vi "Demap symbols.vi"(7 "Symbols":cdb[](array[numeric]) format="%.2f", 9 "Symbol Map":cdb[](array[numeric]) format="%.3f") -> (3 "Output Bit Stream":i8[](array[numeric]))   [LabVIEW 2011]
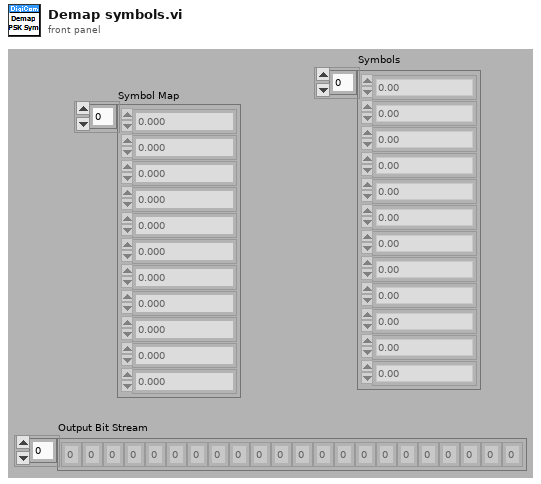
[diagram p1: front panel]
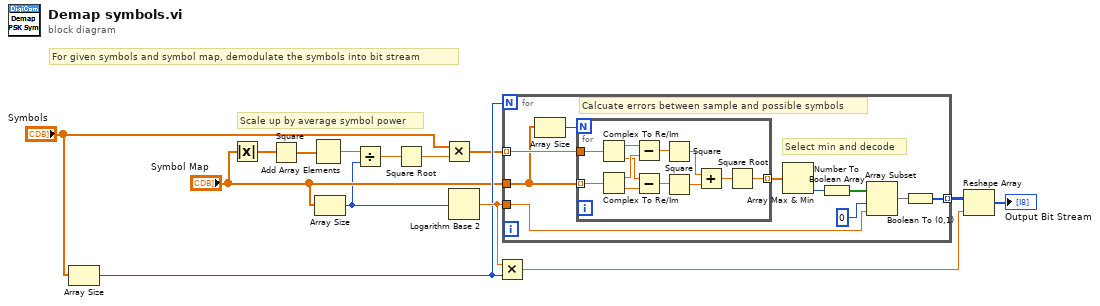
[diagram p0: block diagram]
diagram:
  # "Scale up by average symbol power"
  # "For given symbols and symbol map, demodulate the symbols into bit stream"
  n1 = Array Size(array="Symbols") -> (size(s)=w11:i32)
  n2 = Absolute Value(x="Symbol Map") -> (abs(x)=w8:dbl[])
  n3 = Square(x=w8) -> (x^2=w7:dbl[])
  n4 = Add Array Elements(numeric array=w7) -> (sum=w6:dbl)
  n5 = Array Size(array="Symbol Map") -> (size(s)=w5:i32)
  n6 = Divide(x=w6, y=w5) -> (x/y=w2:dbl)
  n7 = Square Root(x=w2) -> (sqrt(x)=w3:dbl)
  n8 = Multiply(x="Symbols", y=w3) -> (x*y=w1:cdb[])
  n9 = Logarithm Base 2(1:w5) -> (0:w12:dbl)
  n10 = Multiply(x=w12, y=w11) -> (x*y=w10:dbl)
  n11 = for {
    N: w11 -> [_]
    tunnel: w1 -> [w19] mode=indexing
    tunnel: "Symbol Map" -> [w18]
    tunnel: w12 -> [w21]
    tunnel: [w15] -> w14 mode=indexing
    # "Select min and decode"
    # "Calcuate errors between sample and possible symbols"
    n12 = Array Size(array=w18) -> (size(s)=w20:i32)
    n13 = for {
      N: w20 -> [_]
      tunnel: w19 -> [w36]
      tunnel: w18 -> [w35] mode=indexing
      tunnel: [w25] -> w17 mode=indexing
      n14 = Complex To Re/Im(x + iy=w36) -> (x=w34:dbl, y=w32:dbl)
      n15 = Complex To Re/Im(x + iy=w35) -> (x=w33:dbl, y=w31:dbl)
      n16 = Subtract(x=w34, y=w33) -> (x-y=w30:dbl)
      n17 = Subtract(x=w32, y=w31) -> (x-y=w29:dbl)
      n18 = Square(x=w30) -> (x^2=w27:dbl)
      n19 = Square(x=w29) -> (x^2=w28:dbl)
      n20 = Add(x=w27, y=w28) -> (x+y=w26:dbl)
      n21 = Square Root(x=w26) -> (sqrt(x)=w25:dbl)
    }
    n22 = Array Max & Min(array=w17) -> (min index (indices)=w16:i32)  [unwired: 3 out]
    n23 = Number To Boolean Array(number=w16) -> (Boolean array=w24:bool[])
    n24 = Array Subset(array=w24, index=0, length=w21) -> (w22:bool[])
    n25 = Boolean To (0,1)(Boolean=w22) -> (0, 1=w15:i16[])
  }
  n26 = Reshape Array(w14, w10) -> (→"Output Bit Stream":i16[])
